vi "Parse Response Message.vi"(8 "error in":errorcluster, 11 "MPLab in":refnum<class "MPLab.lvclass">) -> (0 "error out":errorcluster, 3 "MPLab out":refnum<class "MPLab.lvclass">)   [LabVIEW 2018, in "MPLab.lvlib" / "MPLab.lvclass"]
uses:
  MPLab.lvclass
  MPLab.lvclass/MPLab.ctl
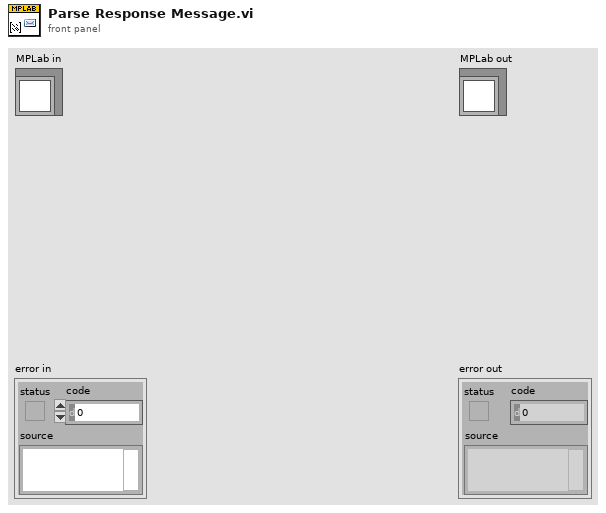
[diagram p1: front panel]
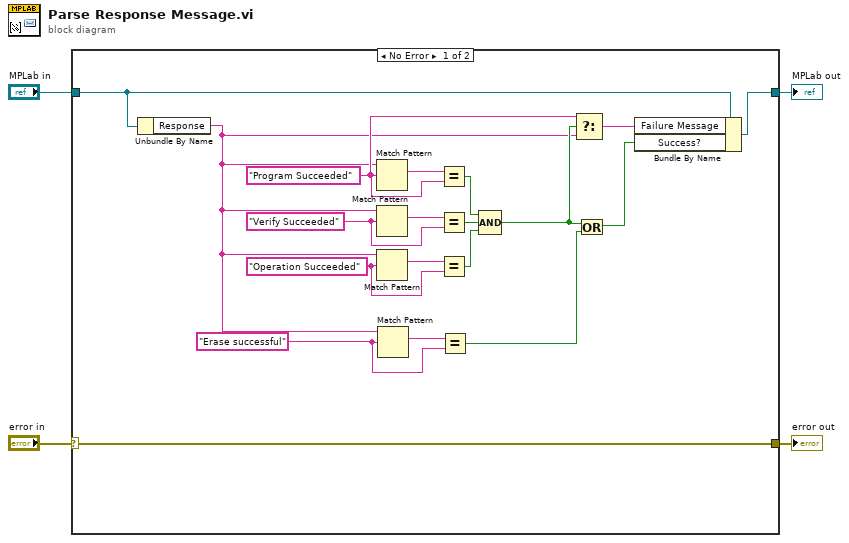
[diagram p0: block diagram]
diagram:
  n1 = case shown="No Error" "error in" {
    selector: "error in" -> [w23 w25]
    tunnel: [w23 w25] -> w1
    tunnel: "MPLab in" -> [w15 w24]
    tunnel: [w14 w24] -> w3
    frame No Error {
      w5 = "Erase successful" ("regular expression")
      w18 = "Operation Succeeded" ("regular expression")
      w21 = "Verify Succeeded" ("regular expression")
      w13 = "Program Succeeded" ("regular expression")
      n2 = Unbundle By Name(w15) -> ("Response"=w7:string)
      n3 = Match Pattern(string=w7, regular expression=w13) -> (match substring=w22:string)  [unwired: 1 in, 3 out]
      n4 = Match Pattern(string=w7, regular expression=w21) -> (match substring=w20:string)  [unwired: 1 in, 3 out]
      n5 = Match Pattern(string=w7, regular expression=w18) -> (match substring=w19:string)  [unwired: 1 in, 3 out]
      n6 = Match Pattern(string=w7, regular expression=w5) -> (match substring=w8:string)  [unwired: 1 in, 3 out]
      n7 = Equal?(x=w22, y=w13) -> (x = y?=w17:bool)
      n8 = Equal?(x=w20, y=w21) -> (x = y?=w16:bool)
      n9 = Equal?(x=w19, y=w18) -> (x = y?=w9:bool)
      n10 = Equal?(x=w8, y=w5) -> (x = y?=w6:bool)
      n11 = Compound Arithmetic op=AND(w17, w16, w9) -> (w10:bool)
      n12 = Select(t=w13, s=w10, f=w7) -> (s? t:f=w12:string)
      n13 = Or(x=w10, y=w6) -> (x .or. y?=w11:bool)
      n14 = Bundle By Name(cluster=w15, "Failure Message"=w12, "Success?"=w11) -> (w14:refnum<class "MPLab.lvclass">)
    }
    frame Error {
    }
  }
  "error out" <- w1
  "MPLab out" <- w3
